vi "Periodic Tasks.vi"(8 "error in":errorcluster) -> ()   [LabVIEW 2015]
doc: "This VI runs in parallel to other tasks. It can contain as many user-defined periodic loops as you need. These can carry out PID or other sorts of timed response."
uses:
  <vilib>/Rock Robotics/WPI/Solenoid/Deprecated/WPI_SolenoidSetBool.vi
  <vilib>/Rock Robotics/WPI/Solenoid/Deprecated/WPI_SolenoidGetBool.vi
  <vilib>/addons/control/pid/pid.llb/PID Output Rate Limiter (DBL).vi
  <vilib>/Rock Robotics/WPI/Utilities/WPI_GetSetVariantRefNum.vi
  <vilib>/addons/control/pid/NI_PID_pid.lvlib
panel:
  in  "dt (s)":dbl=2.0 format="%.2f"
  in  "output rate (EGU/min)":dbl=25.0 format="%.2f"
  in  "initial output":dbl format="%.2f"
  in  "Check PDP/CAN":bool
  out "Bus Off Count":u32
  in  "Check Devices":bool
  out "Device Numbers":u8[](array[numeric])
  out "PDP 3":dbl
  out "PDP 2":dbl
  out "PDP 1":dbl
  out "PDP 0":dbl
  out "Angle":dbl
  in  "Left Art":dbl=0.5 format="%#_13g"
  in  "Right Art":dbl=0.5 format="%#_13g"
  in  "velocity_lower":dbl=1.0 format="%#_13g"
  in  "velocity_upper":dbl=1.0 format="%#_13g"
  out "error out":errorcluster
  # "change in time in milliseconds"
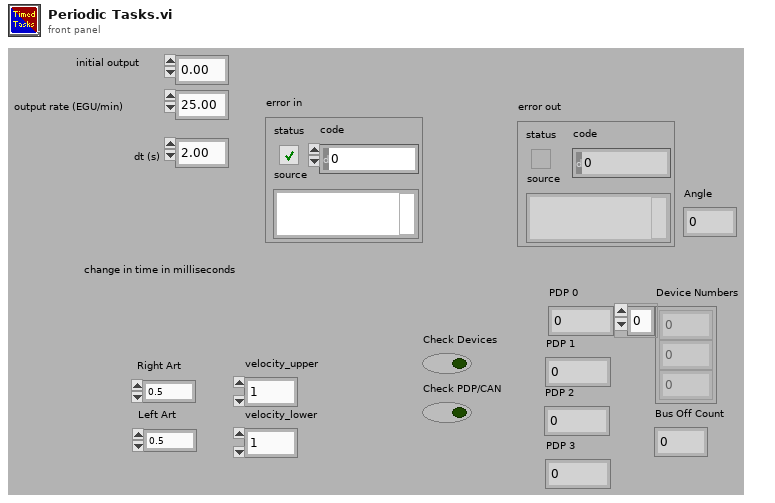
[diagram p1: front panel]
types:
  T1 = typedef "WPI_DigitalInputDevRef.ctl" = cluster{"DevStatus":errorcluster, "DIO Channel":T2}
  T2 = typedef "FPGA_DIOChannel.ctl" = enum8{"DIO 0", "DIO 1", "DIO 2", "DIO 3", "DIO 4", "DIO 5", "DIO 6", "DIO 7", "DIO 8", "DIO 9", "DIO MXP 0", "DIO MXP 1", "DIO MXP 2", "DIO MXP 3", "DIO MXP 4", "DIO MXP 5", "DIO MXP 6", "DIO MXP 7", "DIO MXP 8", "DIO MXP 9", "DIO MXP 10", "DIO MXP 11", "DIO MXP 12", "DIO MXP 13", "DIO MXP 14", "DIO MXP 15", "Invalid"}
  T3 = typedef "WPI_MotorControlDeviceRef.ctl" = cluster{"DeviceStatus":errorcluster, "Type":T4, "PWM":cluster{"PWM Channel":T5, "DeadBand":T6}, "CAN":cluster{"Device Number":u8, "Control Mode":T7, "Semaphore":T8, "Max Vout":dbl, "TalonSRX Control Mode":T9}, "Invert":bool}
  T4 = typedef "WPI_MotorControlType.ctl" = enum16{"PWM", "CAN", "CANTalonSRX"}
  T5 = typedef "FPGA_DIOPWMChannel.ctl" = enum8{"PWM 0", "PWM 1", "PWM 2", "PWM 3", "PWM 4", "PWM 5", "PWM 6", "PWM 7", "PWM 8", "PWM 9", "PWM MXP 0", "PWM MXP 1", "PWM MXP 2", "PWM MXP 3", "PWM MXP 4", "PWM MXP 5", "PWM MXP 6", "PWM MXP 7", "PWM MXP 8", "PWM MXP 9", "Invalid"}
  T6 = typedef "WPI_PWMDeadband.ctl" = cluster{"Name":string, "maxPositivePwm":i32, "minPositivePwm":i32, "centerPwm":i32, "maxNegativePwm":i32, "minNegativePwm":i32, "angularRange":u16}
  T7 = typedef "WPI_CANJaguar_ControlMode.ctl" = enum8{"Percent VBus", "Current", "Speed", "Position", "Voltage"}
  T8 = typedef "Semaphore RefNum" = refnum<k1>
  T9 = typedef "WPI_CANTalonSRX_APIControlMode.ctl" = enum8{"Percent VBus", "Speed", "Position", "Slave", "Unchanged / Invalid", "Voltage Compensation", "Current", "Motion Profile"}
  T10 = typedef "WPI_EncoderDevRef.ctl" = cluster{"DevStatus":errorcluster, "EncoderIndex":T11, "CounterIndex":T12, "DistancePerCount":dbl, "Decoding Type":T13}
  T11 = typedef "FPGA_EncoderIdx.ctl" = enum8{"Enc 0", "Enc 1", "Enc 2", "Enc 3", "Enc 4", "Enc 5", "Enc 6", "Enc 7", "Invalid"}
  T12 = typedef "FPGA_CounterCtrSystemIndex.ctl" = enum8{"Ctr 0", "Ctr 1", "Ctr 2", "Ctr 3", "Ctr 4", "Ctr 5", "Ctr 6", "Ctr 7", "Invalid"}
  T13 = typedef "WPI_EncoderType.ctl" = enum16{"1x", "2x", "4x"}
  T14 = typedef "WPI_GyroDevRef.ctl" = cluster{"DevStatus":errorcluster, "Analog Channel":T15, "Offset":dbl, "Gain (VoltsPerDegree/Second)":dbl, "Gyro Type":enum16{"Analog", "XRS450"}, "Handle":i32, "SPI Bus":T16, "Device Found":bool, "Sample Rate":dbl, "Calibrate On Open":bool}
  T15 = typedef "FPGA_AIChannel.ctl" = enum8{"AI 0", "AI 1", "AI 2", "AI 3", "AI MXP 0", "AI MXP 1", "AI MXP 2", "AI MXP 3", "Invalid"}
  T16 = typedef "spi_bus.ctl" = enum16{"SPI On-Board, CS0", "SPI On-Board, CS1", "SPI On-Board, CS2", "SPI On-Board, CS3", "SPI MXP", "Invalid"}
  T17 = typedef "WPI_DriverStationRobotMode2.ctl" = enum16{"Autonomous Disabled", "Autonomous Enabled", "Teleop Disabled", "Teleop Enabled", "Disconnected", "Finish", "Test Disabled", "Test Enabled", "Emergency Stopped"}
  T18 = typedef "WPI_SolenoidDevRef.ctl" = cluster{"DevStatus":errorcluster, "Pneumatics Control Module":u8, "Forward Solenoid Channel":T19, "Reverse Solenoid Channel":T19}
  T19 = typedef "WPI_SolenoidChannel.ctl" = enum8{"Solenoid 0", "Solenoid 1", "Solenoid 2", "Solenoid 3", "Solenoid 4", "Solenoid 5", "Solenoid 6", "Solenoid 7", "Invalid"}
  T20 = typedef "WPI_RobotDriveDevRef.ctl" = cluster{"DevStatus":errorcluster, "Motors[]":T3[], "Square Inputs":bool, "Max Output":dbl}
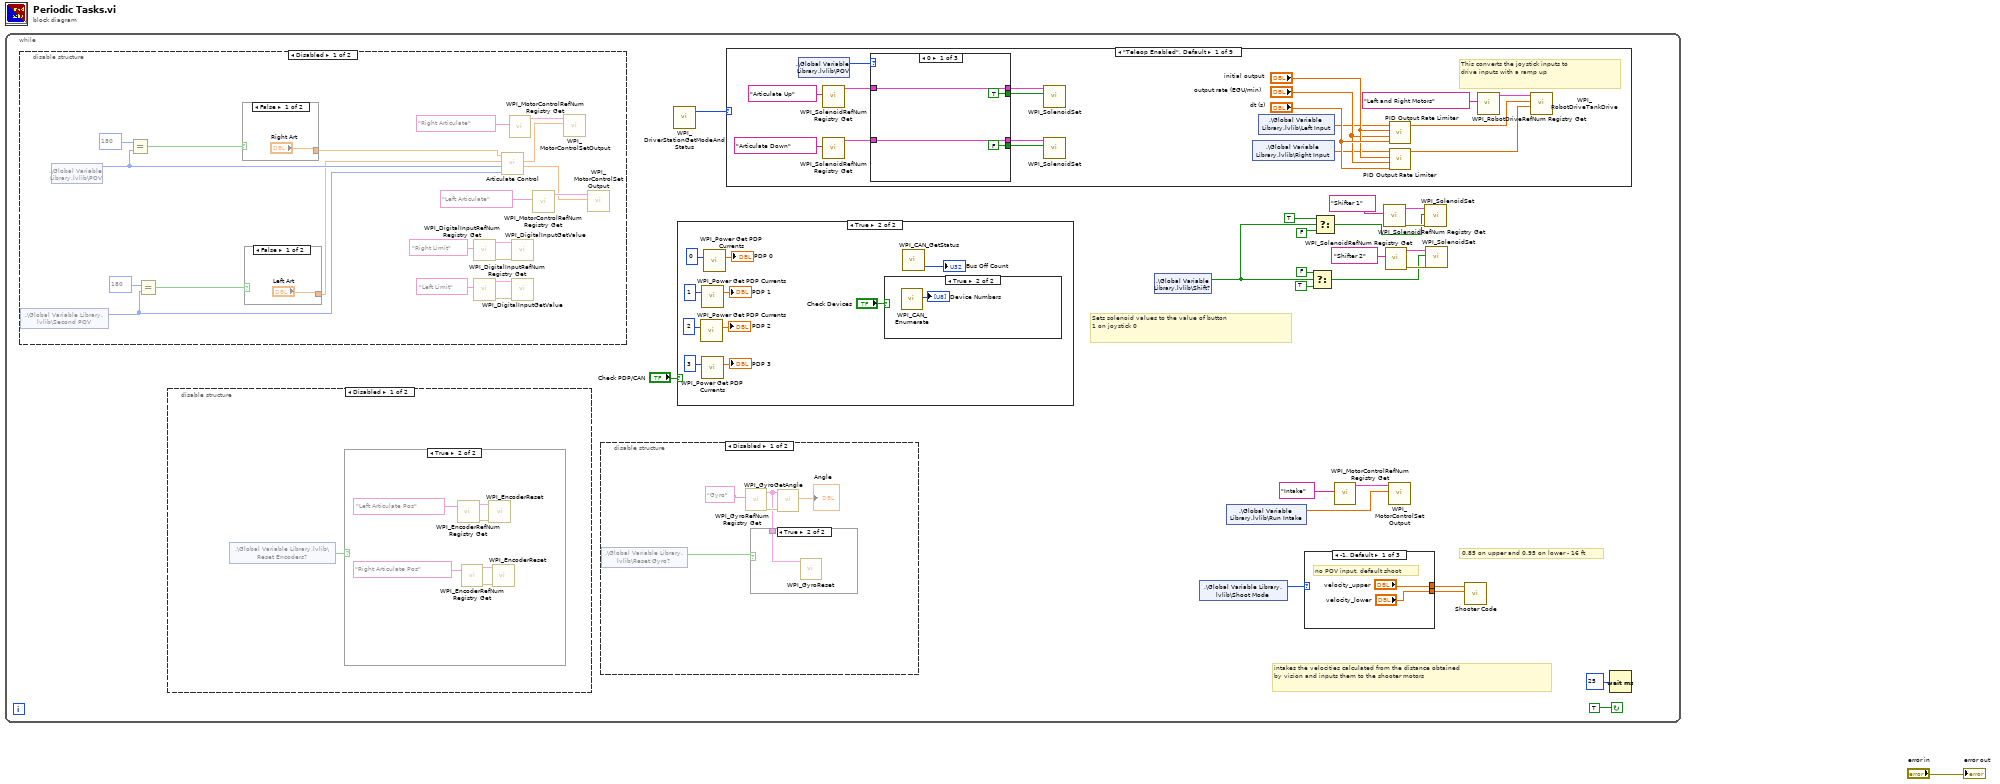
[diagram p0: block diagram]
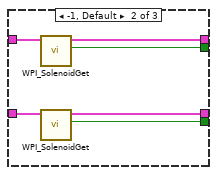
[diagram p4: hidden frame]
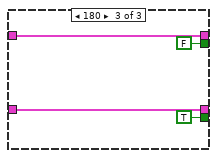
[diagram p5: hidden frame]
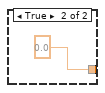
[diagram p18: hidden frame]
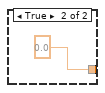
[diagram p19: hidden frame]
diagram:
  n1 = while {
    stop <- TRUE continue-if-true
    # "0.85 on upper and 0.95 on lower - 16 ft"
    # "intakes the velocities calculated from the distance obtained\nby vision and inputs them to the shooter motors"
    # "Sets solenoid values to the value of button\n1 on joystick 0"
    n2 = disable-structure shown="Disabled" {
      frame Disabled {
        n3 = shared-variable ".\\Global Variable Library.lvlib\\Second POV"() -> (w97:i16)  [unwired: 1 in, 1 out]
        n4 = shared-variable ".\\Global Variable Library.lvlib\\POV"() -> (w92:i16)  [unwired: 1 in, 1 out]
        n5 = Equal?(x=i16 180, y=w92) -> (x = y?=w91:bool)
        n6 = Equal?(x=i16 180, y=w97) -> (x = y?=w96:bool)
        n7 = case shown="False" w91 {
          tunnel: ["Right Art" 0.0] -> w93
          frame False {
          }
          frame True {
          }
        }
        n8 = case shown="False" w96 {
          tunnel: ["Left Art" 0.0] -> w87
          frame False {
          }
          frame True {
          }
        }
        n9 = call <vilib>:"WPI_DigitalInputRefNum Registry Get.vi"("refnum name"="Right Limit") -> ("error out"=w81:errorcluster, "DigitalInputDevRef"=w82:T1)  [unwired: 9 in]
        n10 = call <vilib>:"WPI_DigitalInputRefNum Registry Get.vi"("refnum name"="Left Limit") -> ("error out"=w86:errorcluster, "DigitalInputDevRef"=w85:T1)  [unwired: 9 in]
        n11 = call "Articulate Control.vi"("Second POV"=w97, "POV"=w92, "Left Articulate Target"=w87, "Right Articulate Target"=w93) -> ("Left Art Output"=w88:dbl, "Right Art Output"=w95:dbl)  [unwired: 6 in]
        n12 = call <vilib>:"WPI_MotorControlRefNum Registry Get.vi"("refnum name"="Right Articulate") -> ("MotorControlDevRef"=w90:T3)  [unwired: 9 in, 1 out]
        n13 = call <vilib>:"WPI_DigitalInputGetValue.vi"("error in (no error)"=w81, "DigitalInputDevRef"=w82) -> ()  [unwired: 7 in, 3 out]
        n14 = call <vilib>:"WPI_DigitalInputGetValue.vi"("error in (no error)"=w86, "DigitalInputDevRef"=w85) -> ()  [unwired: 7 in, 3 out]
        n15 = call <vilib>:"WPI_MotorControlRefNum Registry Get.vi"("refnum name"="Left Articulate") -> ("MotorControlDevRef"=w99:T3)  [unwired: 9 in, 1 out]
        n16 = call <vilib>:"WPI_MotorControlSetOutput.vi"("Output"=w95, "MotorControlDevRef"=w90) -> ()  [unwired: 7 in, 3 out]
        n17 = call <vilib>:"WPI_MotorControlSetOutput.vi"("Output"=w88, "MotorControlDevRef"=w99) -> ()  [unwired: 7 in, 3 out]
      }
      frame Enabled {
      }
    }
    n18 = disable-structure shown="Disabled" {
      frame Disabled {
        n19 = shared-variable ".\\Global Variable Library.lvlib\\Reset Encoders?"() -> (w74:bool)  [unwired: 1 in, 1 out]
        n20 = case shown="True" w74 {
          frame False {
          }
          frame True {
            n21 = call <vilib>:"WPI_EncoderRefNum Registry Get.vi"("refnum name"="Left Articulate Pos") -> ("error out"=w80:errorcluster, "EncoderDevRef"=w79:T10)  [unwired: 9 in]
            n22 = call <vilib>:"WPI_EncoderRefNum Registry Get.vi"("refnum name"="Right Articulate Pos") -> ("error out"=w75:errorcluster, "EncoderDevRef"=w76:T10)  [unwired: 9 in]
            n23 = call <vilib>:"WPI_EncoderReset.vi"("error in (no error)"=w80, "EncoderDevRef"=w79) -> ()  [unwired: 8 in, 2 out]
            n24 = call <vilib>:"WPI_EncoderReset.vi"("error in (no error)"=w75, "EncoderDevRef"=w76) -> ()  [unwired: 8 in, 2 out]
          }
        }
      }
      frame Enabled {
      }
    }
    n25 = disable-structure shown="Disabled" {
      frame Disabled {
        n26 = shared-variable ".\\Global Variable Library.lvlib\\Reset Gyro?"() -> (w68:bool)  [unwired: 1 in, 1 out]
        n27 = call <vilib>:"WPI_GyroRefNum Registry Get.vi"("refnum name"="Gyro") -> ("error out"=w72:errorcluster, "GyroDevRef"=w69:T14)  [unwired: 9 in]
        n28 = case shown="True" w68 {
          tunnel: w69 -> [_ w73]
          frame False {
          }
          frame True {
            n29 = call <vilib>:"WPI_GyroReset.vi"("GyroDevRef"=w73) -> ()  [unwired: 9 in, 2 out]
          }
        }
        n30 = call <vilib>:"WPI_GyroGetAngle.vi"("error in"=w72, "GyroDevRef"=w69) -> ("Angle"=→"Angle":dbl)  [unwired: 5 in, 4 out]
      }
      frame Enabled {
      }
    }
    n31 = call <vilib>:"WPI_DriverStationGetModeAndStatus.vi"() -> ("Robot Mode"=w3:T17)  [unwired: 10 in, 1 out]
    n32 = case shown="True" "Check PDP/CAN" {
      frame False {
      }
      frame True {
        n33 = call <vilib>:"WPI_Power Get PDP Currents.vi"("PDP Channel"=2) -> ("current (A)"=→"PDP 2":dbl)  [unwired: 12 in, 2 out]
        n34 = call <vilib>:"WPI_Power Get PDP Currents.vi"("PDP Channel"=1) -> ("current (A)"=→"PDP 1":dbl)  [unwired: 12 in, 2 out]
        n35 = call <vilib>:"WPI_Power Get PDP Currents.vi"("PDP Channel"=3) -> ("current (A)"=→"PDP 3":dbl)  [unwired: 12 in, 2 out]
        n36 = call <vilib>:"WPI_Power Get PDP Currents.vi"("PDP Channel"=0) -> ("current (A)"=→"PDP 0":dbl)  [unwired: 12 in, 2 out]
        n37 = case shown="True" "Check Devices" {
          frame False {
          }
          frame True {
            n38 = call <vilib>:"WPI_CAN_Enumerate.vi"() -> ("Device Numbers"=→"Device Numbers":u8[])  [unwired: 10 in, 1 out]
          }
        }
        n39 = call <vilib>:"WPI_CAN_GetStatus.vi"() -> ("Bus Off Count"=→"Bus Off Count":u32)  [unwired: 6 in, 5 out]
      }
    }
    n40 = case shown="\"Teleop Enabled\", Default" w3 {
      frame "Teleop Enabled", Default {
        # "This converts the joystick inputs to\ndrive inputs with a ramp up"
        n41 = shared-variable ".\\Global Variable Library.lvlib\\POV"() -> (w53:i16)  [unwired: 1 in, 1 out]
        n42 = call <vilib>:"WPI_SolenoidRefNum Registry Get.vi"("refnum name"="Articulate Up") -> ("SolenoidDevRef"=w45:T18)  [unwired: 9 in, 1 out]
        n43 = call <vilib>:"WPI_SolenoidRefNum Registry Get.vi"("refnum name"="Articulate Down") -> ("SolenoidDevRef"=w52:T18)  [unwired: 9 in, 1 out]
        n44 = case shown="0" w53 {
          tunnel: w52 -> [w57 w63 w65]
          tunnel: [w57 w62 w65] -> w51
          tunnel: [FALSE ("Value") w61 TRUE ("Value")] -> w50
          tunnel: w45 -> [w56 w58 w66]
          tunnel: [w56 w59 w66] -> w46
          tunnel: [TRUE ("Value") w60 FALSE ("Value")] -> w47
          frame 0 {
          }
          frame -1, Default {
            n45 = call-poly <vilib>:"WPI_SolenoidGet.vi"("SolenoidDevRef"=w58) -> ("Value"=w60:bool, "SolenoidDevRef"=w59:T18)  [unwired: 8 in, 1 out]
            n46 = call-poly <vilib>:"WPI_SolenoidGet.vi"("SolenoidDevRef"=w63) -> ("Value"=w61:bool, "SolenoidDevRef"=w62:T18)  [unwired: 8 in, 1 out]
          }
          frame 180 {
          }
        }
        n47 = call-poly <vilib>:"WPI_SolenoidSet.vi"("Value"=w47, "SolenoidDevRef"=w46) -> ()  [unwired: 8 in, 2 out]
        n48 = call-poly <vilib>:"WPI_SolenoidSet.vi"("Value"=w50, "SolenoidDevRef"=w51) -> ()  [unwired: 8 in, 2 out]
        n49 = shared-variable ".\\Global Variable Library.lvlib\\Right Input"() -> (w36:dbl)  [unwired: 1 in, 1 out]
        n50 = shared-variable ".\\Global Variable Library.lvlib\\Left Input"() -> (w37:dbl)  [unwired: 1 in, 1 out]
        n51 = call-poly <vilib>:"PID Output Rate Limiter.vi"("dt (s)"="dt (s)", "output rate (EGU/min)"="output rate (EGU/min)", "initial output"="initial output", "input (controller output)"=w37) -> ("output"=w44:dbl)  [unwired: 4 in, 1 out]
        n52 = call-poly <vilib>:"PID Output Rate Limiter.vi"("dt (s)"="dt (s)", "output rate (EGU/min)"="output rate (EGU/min)", "initial output"="initial output", "input (controller output)"=w36) -> ("output"=w40:dbl)  [unwired: 4 in, 1 out]
        n53 = call <vilib>:"WPI_RobotDriveRefNum Registry Get.vi"("refnum name"="Left and Right Motors") -> ("RobotDriveDevRef"=w42:T20)  [unwired: 9 in, 1 out]
        n54 = call <vilib>:"WPI_RobotDriveTankDrive.vi"("Right axis value"=w40, "Left axis value"=w44, "RobotDriveDevRef"=w42) -> ()  [unwired: 6 in, 3 out]
      }
      frame "Disconnected" {
      }
      frame "Finish" {
      }
      frame "Test Disabled" {
      }
      frame "Test Enabled" {
      }
      frame "Emergency Stopped" {
      }
      frame "Teleop Disabled" {
      }
      frame "Autonomous Enabled" {
      }
      frame "Autonomous Disabled" {
      }
    }
    n55 = shared-variable ".\\Global Variable Library.lvlib\\Shift?"() -> (w10:bool)  [unwired: 1 in, 1 out]
    n56 = shared-variable ".\\Global Variable Library.lvlib\\Shoot Mode"() -> (w5:i16)  [unwired: 1 in, 1 out]
    n57 = shared-variable ".\\Global Variable Library.lvlib\\Run Intake"() -> (w4:dbl)  [unwired: 1 in, 1 out]
    n58 = case shown="-1, Default" w5 {
      tunnel: ["velocity_upper" w108 w110] -> w7
      tunnel: ["velocity_lower" w107 w109] -> w6
      frame -1, Default {
        # "no POV input, default shoot"
      }
      frame 0 {
        w107 = 1.0  # velocity_lower
        w108 = 1.0  # velocity_upper
        # "far shot, north direction"
      }
      frame 180 {
        w109 = 0.5  # velocity_lower
        w110 = 0.5  # velocity_upper
        # "short shot south direction"
      }
    }
    n59 = Select(t=FALSE ("f"), s=w10, f=TRUE) -> (s? t:f=w11:bool)
    n60 = Select(t=TRUE, s=w10, f=FALSE) -> (s? t:f=w12:bool)
    n61 = call <vilib>:"WPI_MotorControlRefNum Registry Get.vi"("refnum name"="Intake") -> ("MotorControlDevRef"=w8:T3)  [unwired: 9 in, 1 out]
    n62 = call <vilib>:"WPI_SolenoidRefNum Registry Get.vi"("refnum name"="Shifter 1") -> ("error out"=w20:errorcluster, "SolenoidDevRef"=w19:T18)  [unwired: 9 in]
    n63 = call <vilib>:"WPI_SolenoidRefNum Registry Get.vi"("refnum name"="Shifter 2") -> ("error out"=w18:errorcluster, "SolenoidDevRef"=w17:T18)  [unwired: 9 in]
    n64 = call <vilib>:"WPI_MotorControlSetOutput.vi"("Output"=w4, "MotorControlDevRef"=w8) -> ()  [unwired: 7 in, 3 out]
    n65 = call-poly <vilib>:"WPI_SolenoidSet.vi"("error in (no error)"=w20, "Value"=w12, "SolenoidDevRef"=w19) -> ()  [unwired: 7 in, 2 out]
    n66 = call-poly <vilib>:"WPI_SolenoidSet.vi"("error in (no error)"=w18, "Value"=w11, "SolenoidDevRef"=w17) -> ()  [unwired: 7 in, 2 out]
    n67 = call "Shooter Code.vi"("velocity_lower"=w6, "velocity_upper"=w7) -> ()  [unwired: 10 in]
    n68 = Wait (ms)(milliseconds to wait=u32 25) -> ()  [unwired: 1 out]
  }
  "error out" <- "error in"
